vi "Read Digital Output.vi"(8 "error in (no error)":errorcluster, 11 "DAQmx Watchdog configuration in":refnum<class "DAQmx Watchdog configuration.lvclass">) -> (0 "error out":errorcluster, 2 "Digital Output":T1(array[cluster]) {"expiration state" items=["High"=10192, "Low"=10214, "Tristate"=10310, "No Change"=10160]}, 3 "DAQmx Watchdog configuration out":refnum<class "DAQmx Watchdog configuration.lvclass">)   [LabVIEW 2014, in "DAQmx Watchdog configuration.lvclass"]
uses:
  DAQmx Watchdog configuration.lvclass
  DAQmx Watchdog configuration.lvclass/DAQmx Watchdog configuration.ctl
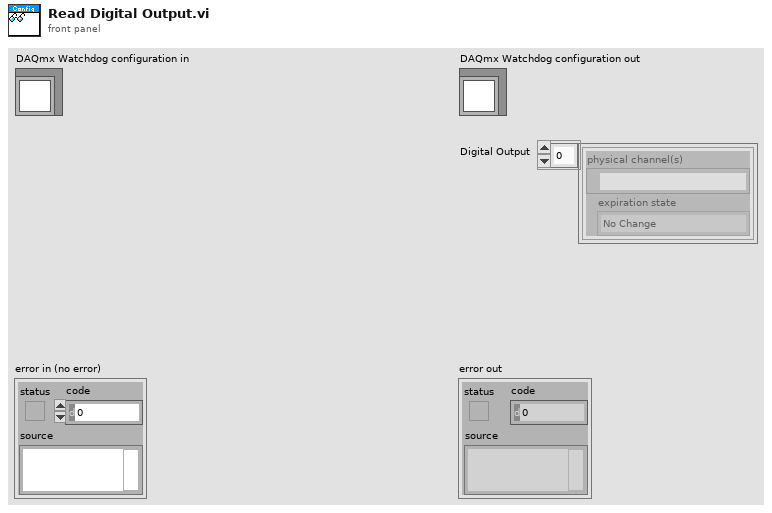
[diagram p1: front panel]
types:
  T1 = cluster{"physical channel(s)":tag, "expiration state":i32}[]
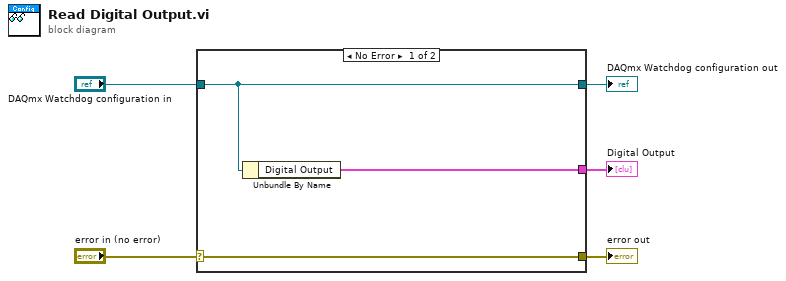
[diagram p0: block diagram]
diagram:
  n1 = case shown="No Error" "error in (no error)" {
    selector: "error in (no error)" -> [w8 w9]
    tunnel: [w8 w9] -> w4
    tunnel: [w7 w10] -> w2
    tunnel: "DAQmx Watchdog configuration in" -> [w7 w10]
    tunnel: [w6 _] -> w1
    frame No Error {
      n2 = Unbundle By Name(w7) -> ("Digital Output"=w6:T1)
    }
    frame Error {
    }
  }
  "error out" <- w4
  "DAQmx Watchdog configuration out" <- w2
  "Digital Output" <- w1
